vi "Read Child Attributes.vi"(7 "Actor in":refnum<class "Actor.lvclass">) -> (2 "Child Attributes":T1)   [LabVIEW 2020, in "jettl.lvlib" / "Actor Specific.lvlib"]
uses:
  Actor Specific.lvlib
  Actor/Actor.lvclass
  Msg/Msg.lvclass
  Transport/Transport.lvclass
  Attributes Metadata/Attributes Metadata.lvclass
  Msgs.ctl
  jettl.lvlib
  Attributes.ctl
  Child Attributes.ctl
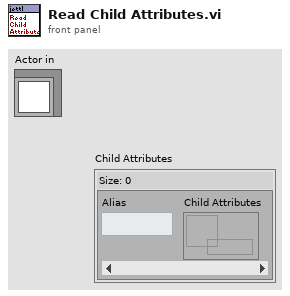
[diagram p1: front panel]
types:
  T1 = typedef "jettl.lvlib/Child Attributes.ctl" = map{string, refnum<data-value>}
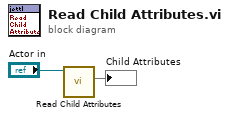
[diagram p0: block diagram]
diagram:
  n1 = call-dynamic "Read Child Attributes.vi"("Actor in"="Actor in") -> ("Child Attributes"=→"Child Attributes":T1)  [unwired: 10 in]
